vi "Read SCH Param File and set FPGA MGI RWA.vi"(8 "error in (no error)":errorcluster, 11 "FPGA Refnum in":T2) -> (0 "error out":errorcluster, 2 "FPGA Configuration Values":T1={"Ln2 Filter Size"=10, "VT Quench Tick Limit"=4000000, "VT Quench Volt Limit"=0.100006103515625, "Joint Tick Limit"=4000000, "Joint Volt Limit"=0.00020000338554382324, "CoWound Volt Limit"=0.20001220703125, "CoWound Tick Limit"=4000000, "SC Bus Limit"=0.0004000067710876465, "SC Bus Tick Limit"=4000000, "ResMag Tick Limit"=1000000, "DAQ Cycle Ticks"=4096, "Res Mag dI/dt Delay"=256, "dI/dT scaling"=38.14697265625, "Pressure Inlet Limit (BarA)"=6.0, "Bore Tube Volt Limit"=0.5999999940395355, "Pressure Outlet Limit (BarA)"=5.0, "Activation Current (kA)"=0.5, "Dump Resistor Scale Factor"=204.79399999976158, "Co-Wound Asymmetry Factor"=0.0099029541015625, "Co-Wound Scale Factor"=60.04379999637604, "Layer Scale Factors"=[4.000479996204376, 3.5011550039052963, 3.5012779980897903, 3.5011550039052963, 3.001561000943184, 3.001561000943184, 3.5000530034303665, 3.500664994120598, 3.5011550039052963, 4.000159993767738, 3.999679997563362, 4.000159993767738, 3.998879998922348, 3.999520003795624, 3.999679997563362, 4.000320002436638, 4.000960007309914, 4.000640004873276], "Fudge Factors"=[0.0, 0.0, 0.0, 0.0, 0.0, 0.0, 0.0, 0.0, 0.0, 0.0, 0.0, 0.0, 0.0, 0.0, 0.0, 0.0], "Joint Scale Factors"=[0.0002005249261856079, 0.0002005249261856079, 0.00020040571689605713, 0.00020048022270202637, 0.00020040571689605713, 0.00020076334476470947, 0.00020068883895874023, 0.0002006441354751587], "SC Bus Scale"=[0.09999999403953552, 0.09999999403953552, 0.0010000020265579224, 0.0010000020265579224, 0.0002005249261856079, 0.0002006441354751587], "Pressure Scale Factor"=[1.723690003156662, 1.723690003156662, 1.723690003156662, 1.723690003156662], "# Consecutive Zeros Fault"=1000, "Digitize Convert Ticks"=200, "Digitize Reset Ticks"=400, "Convert Clock Ticks"=20, "Digitize Read Delay Ticks"=38, "Digitize # Bits"=16, "HTS Lead Tick Limit"=4000000, "Res Lead Tick Limit"=4000000, "HTS Lead Trip"=0.15000000596046448, "Res Lead Limit"=0.001953125, "HTS Lead FRZ"=0.006999999284744263, "HTS Lead Warn"=0.0010000020265579224, "Low Current (kA)"=0.04500000178813934, "Low Current Ticks"=400000000, "Low Current Delay Factor"=100, "HTS Resistance (nOhm)"=[0.0, 0.0], "Ticks to Close Relief"=80000000, "All Breaker Tick Limit"=400000000, "HTS Offset (microV)"=[0.0, 0.0], "Delay Ticks Between Bkr Reset"=1200000000, "Breaker Reset Ticks"=400000000, "PS Enable Reset Ticks"=400000000, "Reset Digitizer Ticks"=400000000, "Pressure Inlet Cooldown Limit"=12.0, "Pressure Outlet Cooldown Limit"=10.0, "Notification Email"="sth@magnet.fsu.edu"} {"Pressure Outlet Cooldown Limit" format="%.5g"; "Pressure Inlet Cooldown Limit" format="%.5g"; "HTS Offset (microV)" format="%_6g"; "HTS Resistance (nOhm)" format="%_6g"; "HTS Lead Warn" format="%_6g"; "HTS Lead FRZ" format="%_6g"; "Res Lead Limit" format="%_6g"; "HTS Lead Trip" format="%_6g"; "Pressure Scale Factor" format="%_6g"; "Joint Scale Factors" format="%_6g"; "Fudge Factors" format="%.7g"; "Co-Wound Asymmetry Factor" format="%.8g"; "Activation Current (kA)" format="%_6g"; "Pressure Outlet Limit (BarA)" format="%.5g"; "Bore Tube Volt Limit" format="%_6g"; "Pressure Inlet Limit (BarA)" format="%.5g"; "dI/dT scaling" format="%.11g"; "SC Bus Limit" format="%_6g"; "Joint Volt Limit" format="%_6g"; "VT Quench Volt Limit" format="%.5g"}, 3 "Refnum out":T2)   [LabVIEW 2018]
doc: "Author: Scott Hannahs <sth@magnet.fsu.edu>\nCopyright 2018 Florida State University, All rights reserved."
uses:
  RT Controls/FPGA SCH Digitizer Ref.ctl
  SCH Data Controls/FPGA Configure Parameters.ctl
  <userlib>/_MGI/Read Write Anything/MGI RWA Options Cluster.ctl
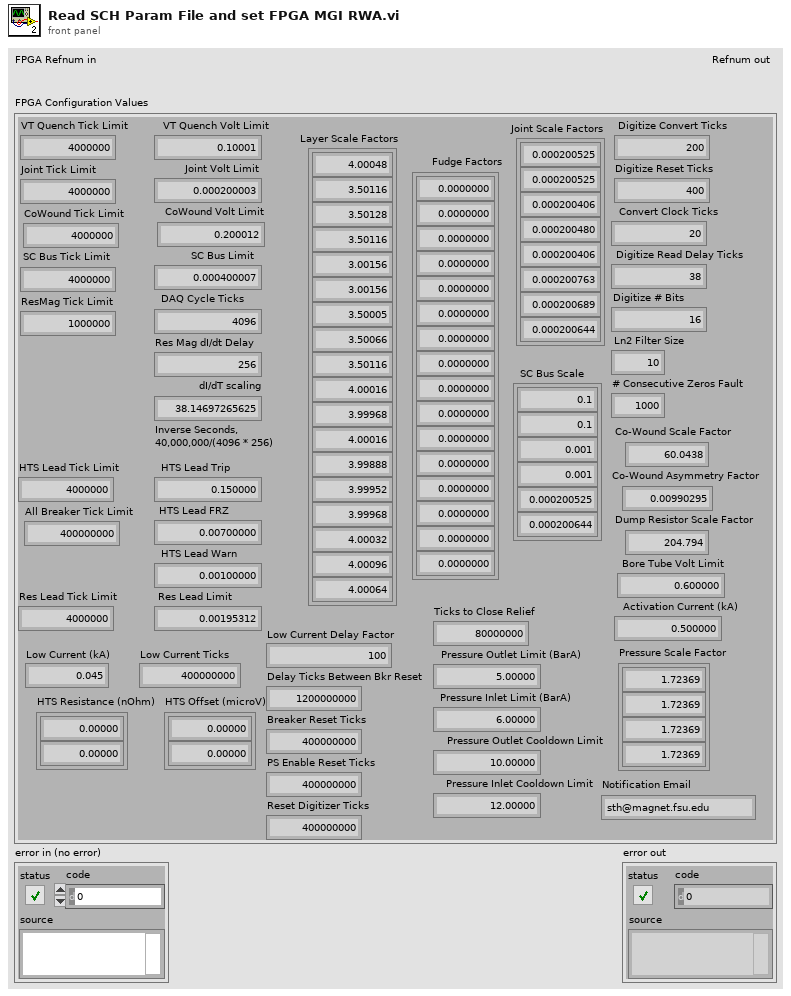
[diagram p1: front panel]
types:
  T1 = typedef "FPGA Configure Parameters.ctl" = cluster{"Ln2 Filter Size":i16, "VT Quench Tick Limit":u32, "VT Quench Volt Limit":dbl, "Joint Tick Limit":u32, "Joint Volt Limit":dbl, "CoWound Volt Limit":dbl, "CoWound Tick Limit":u32, "SC Bus Limit":dbl, "SC Bus Tick Limit":u32, "ResMag Tick Limit":u32, "DAQ Cycle Ticks":u32, "Res Mag dI/dt Delay":u32, "dI/dT scaling":dbl, "Pressure Inlet Limit (BarA)":dbl, "Bore Tube Volt Limit":dbl, "Pressure Outlet Limit (BarA)":dbl, "Activation Current (kA)":dbl, "Dump Resistor Scale Factor":dbl, "Co-Wound Asymmetry Factor":dbl, "Co-Wound Scale Factor":dbl, "Layer Scale Factors":dbl[], "Fudge Factors":dbl[], "Joint Scale Factors":dbl[], "SC Bus Scale":dbl[], "Pressure Scale Factor":dbl[], "# Consecutive Zeros Fault":i16, "Digitize Convert Ticks":u32, "Digitize Reset Ticks":u32, "Convert Clock Ticks":u32, "Digitize Read Delay Ticks":u32, "Digitize # Bits":u32, "HTS Lead Tick Limit":u32, "Res Lead Tick Limit":u32, "HTS Lead Trip":dbl, "Res Lead Limit":dbl, "HTS Lead FRZ":dbl, "HTS Lead Warn":dbl, "Low Current (kA)":dbl, "Low Current Ticks":u32, "Low Current Delay Factor":u16, "HTS Resistance (nOhm)":dbl[], "Ticks to Close Relief":u32, "All Breaker Tick Limit":u32, "HTS Offset (microV)":dbl[], "Delay Ticks Between Bkr Reset":u32, "Breaker Reset Ticks":u32, "PS Enable Reset Ticks":u32, "Reset Digitizer Ticks":u32, "Pressure Inlet Cooldown Limit":dbl, "Pressure Outlet Cooldown Limit":dbl, "Notification Email":string}
  T2 = typedef "FPGA SCH Digitizer Ref.ctl" = refnum<k20>
  T3 = typedef "MGI RWA Options Cluster.ctl" = cluster{"TS Fmt":string, "Int Fmt":string, "Delimiter":string}
  T4 = cluster{"Ln2 Filter Size":i16, "VT Quench Tick Limit":u32, "VT Quench Volt Limit":dbl, "Joint Tick Limit":u32, "Joint Volt Limit":dbl, "CoWound Volt Limit":dbl, "CoWound Tick Limit":u32, "SC Bus Limit":dbl, "SC Bus Tick Limit":u32, "ResMag Tick Limit":u32, "DAQ Cycle Ticks":u32, "Res Mag dI/dt Delay":u32, "dI/dT scaling":dbl, "Pressure Inlet Limit (BarA)":dbl, "Bore Tube Volt Limit":dbl, "Pressure Outlet Limit (BarA)":dbl, "Activation Current (kA)":dbl, "Dump Resistor Scale Factor":dbl, "Co-Wound Asymmetry Factor":dbl, "Co-Wound Scale Factor":dbl, "Layer Scale Factors":dbl[], "Fudge Factors":dbl[], "Joint Scale Factors":dbl[], "SC Bus Scale":dbl[], "Pressure Scale Factor":dbl[], "# Consecutive Zeros Fault":i16, "Digitize Convert Ticks":u32, "Digitize Reset Ticks":u32, "Convert Clock Ticks":u32, "Digitize Read Delay Ticks":u32, "Digitize # Bits":u32, "HTS Lead Tick Limit":u32, "Res Lead Tick Limit":u32, "HTS Lead Trip":dbl, "Res Lead Limit":dbl, "HTS Lead FRZ":dbl, "HTS Lead Warn":dbl, "Low Current (kA)":dbl, "Low Current Ticks":u32, "Low Current Delay Factor":u16, "HTS Resistance (nOhm)":dbl[], "Ticks to Close Relief":u32, "All Breaker Tick Limit":u32, "HTS Offset (microV)":dbl[], "Delay Ticks Between Bkr Reset":u32, "Breaker Reset Ticks":u32, "PS Enable Reset Ticks":u32, "Reset Digitizer Ticks":u32, "Pressure Inlet Cooldown Limit":dbl, "Pressure Outlet Cooldown Limit":dbl, "Notification Email":string}
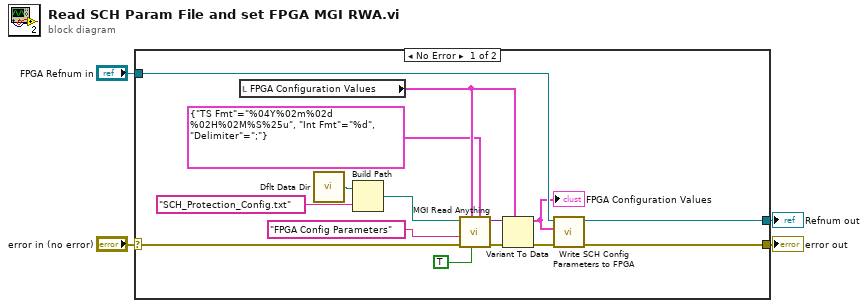
[diagram p0: block diagram]
diagram:
  n1 = case shown="No Error" "error in (no error)" {
    selector: "error in (no error)" -> [w7 w21]
    tunnel: [w15 w21] -> w3
    tunnel: "FPGA Refnum in" -> [w17 w20]
    tunnel: [w16 w20] -> w1
    frame No Error {
      n2 = local read "FPGA Configuration Values"() -> (w12:T1)
      n3 = call <vilib>:"Dflt Data Dir.vi"() -> ("App:Default Data Directory"=w19:path)
      n4 = Build Path(base path=w19, name or relative path="SCH_Protection_Config.txt") -> (appended path=w11:path)
      n5 = call <userlib>:"MGI Read Anything.vi"("Read/Write Options (Version 1.x)"=T3 {"TS Fmt"="%04Y%02m%02d %02H%02M%S%25u", "Int Fmt"="%d", "Delimiter"=";"}, "Use Supplied (F: Use Default)"=TRUE, "Type of Anything"=w12, "Error In"=w7, "Section Name (Name of \"Type of Anything\")"="FPGA Config Parameters" ("section"), "Path (dialog)"=w11) -> ("Error Out"=w14:errorcluster, "Anything"=w13:variant)  [unwired: 2 in, 2 out]
      n6 = Variant To Data(error in=w14, type=w12, Variant=w13) -> (data=w9:T4, error out=w8:errorcluster)
      "FPGA Configuration Values" <- w9
      n7 = call "Write SCH Config Parameters to FPGA.vi"("error in (no error)"=w8, "FPGA Configuration Values"=w9, "Refnum in"=w17) -> ("error out"=w15:errorcluster, "Refnum out"=w16:T2)  [unwired: 7 in]
    }
    frame Error {
    }
  }
  "Refnum out" <- w1
  "error out" <- w3
